vi "Display.vi"(8 "error in (no error)":errorcluster, 11 "DisplayTetrodes in":refnum<class "DisplayTetrodes.lvclass">) -> (0 "error out":errorcluster, 3 "DisplayTetrodes out":refnum<class "DisplayTetrodes.lvclass">)   [LabVIEW 2010, in "DisplayTetrodes.lvclass"]
uses:
  DisplayTetrodes.lvclass
  <vilib>/Analysis/3filter.llb/Filter Passband Type.ctl
  <vilib>/Analysis/2dsp.llb/Decimate (continuous, DBL).vi
  <vilib>/Analysis/3filter.llb/Butterworth Filter (DBL).vi
  Program Files/National Instruments/LabVIEW 2010/resource/objmgr/ni.dex.rc
  <vilib>/Analysis/NI_AALBase.lvlib
  <vilib>/Analysis/NI_AALPro.lvlib
panel:
  in  "Tab Control":enum32{"Connection", "Filter", "Display Params"}(tab)
  in  "Network Stream Writer IP":string(combo)
  out "Connected":bool
  out "Elems Left":i32(slide) scale=0.0..100.0
  in  "High Cutoff (Hz)":dbl=6000.0 format="%0.2f"
  in  "Low Cutoff (Hz)":dbl=600.0 format="%0.4f"
  in  "Filter Type":T1=enum."Bandpass"
  in  "FilterData":bool=TRUE
  in  "Decimation Factor":i32=4
  in  "Spacing":dbl=0.0001
  in  "Scale":dbl=1.0
  in  "DiodeScale":dbl=0.05
  out "Waveform Chart":waveform(dbl)[](graph)
  in  "STOP":bool
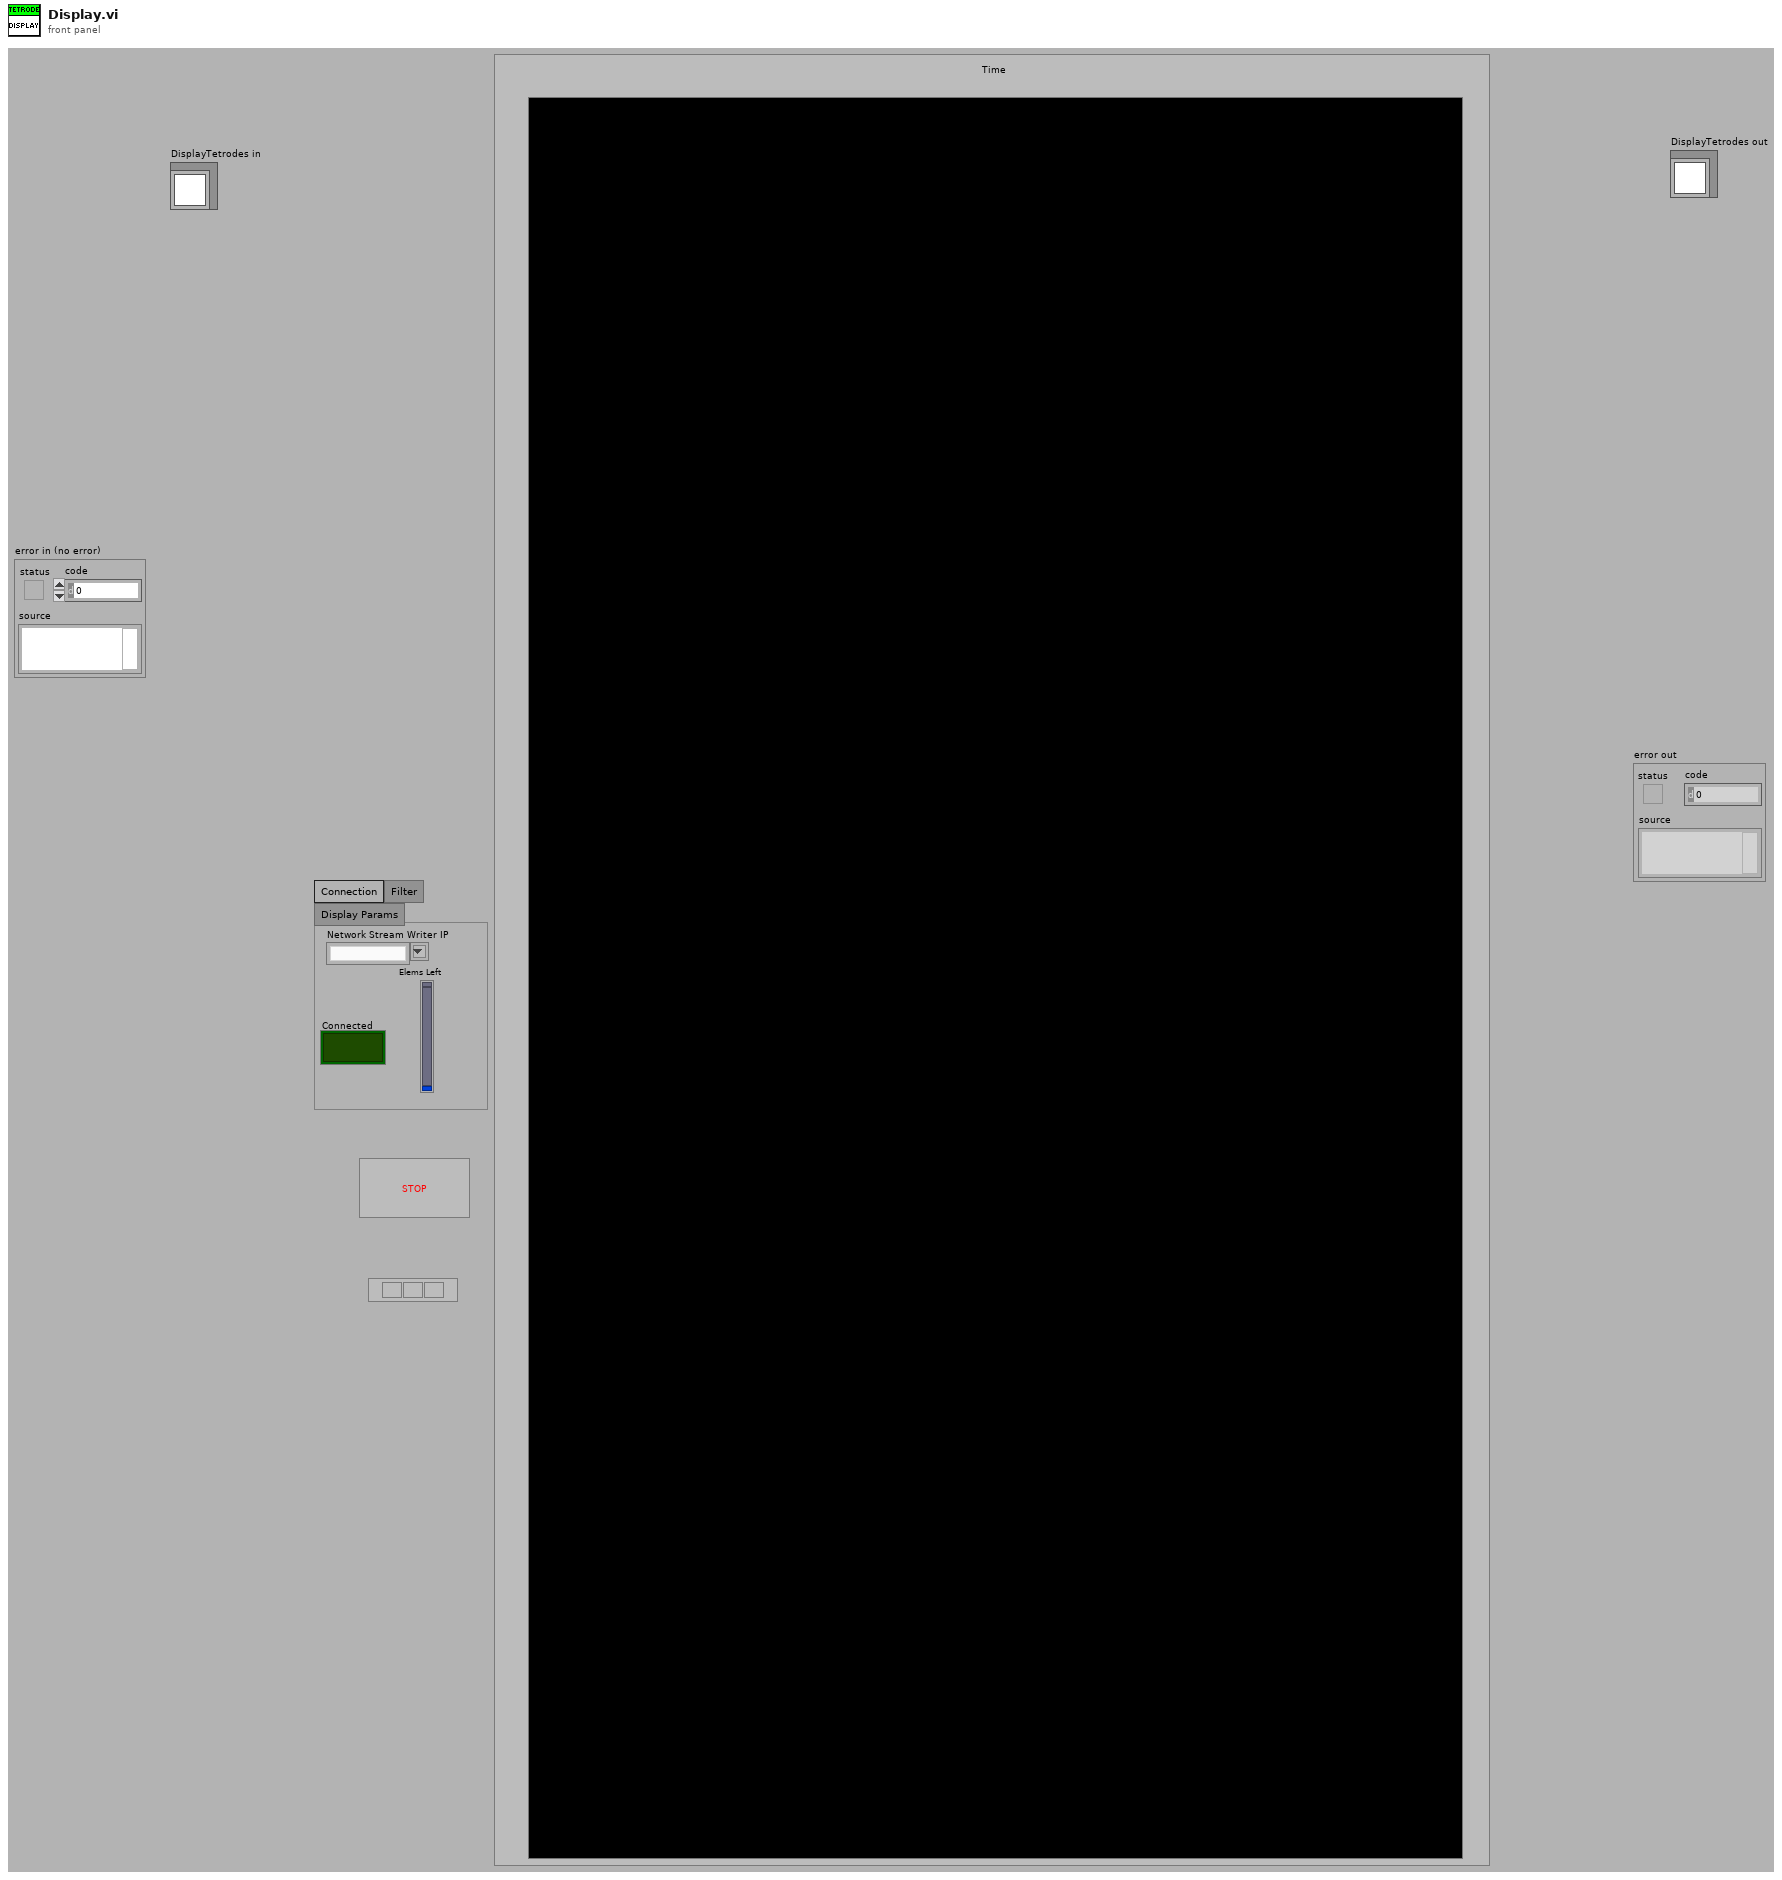
[diagram p1: front panel]
types:
  T1 = typedef "NI_AALBase.lvlib/Filter Passband Type.ctl" = enum32{"Lowpass", "Highpass", "Bandpass", "Bandstop"}
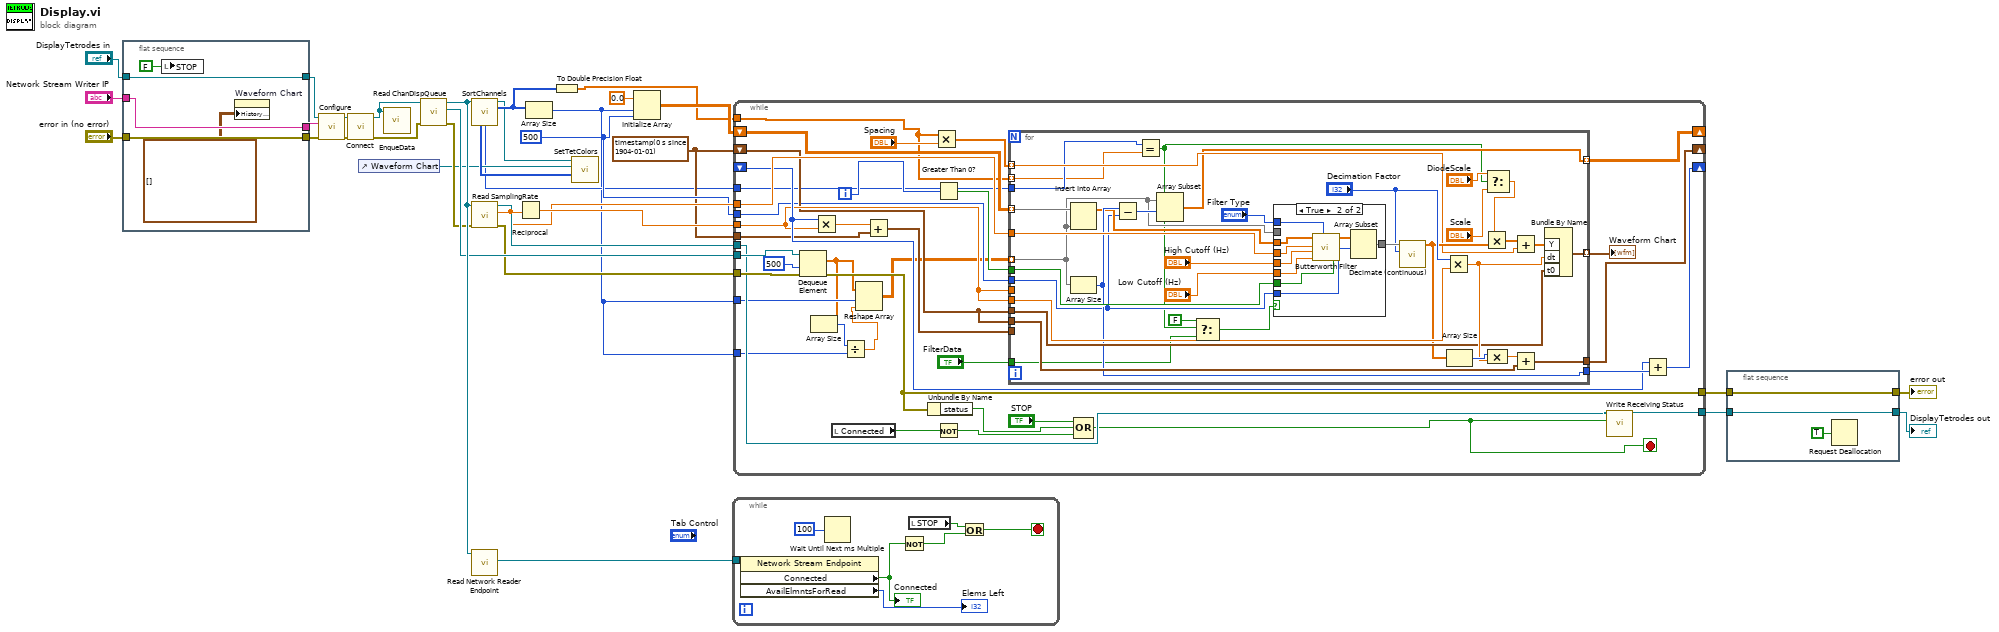
[diagram p0: block diagram]
diagram:
  w8 = timestamp(0 s since 1904-01-01)
  w9 = 500 ("y")
  n1 = flat-sequence {
    tunnel: "DisplayTetrodes in" -> [w37]
    tunnel: [w37] -> w17
    tunnel: "Network Stream Writer IP" -> [w36]
    tunnel: [w36] -> w15
    tunnel: "error in (no error)" -> [w35]
    tunnel: [w35] -> w13
    frame #0 {
      n2 = local write "STOP"(FALSE ("STOP")) -> ()
      n3 = property on="Waveform Chart" class="WFChart (strict)"("History Data"=waveform(dbl)[][] []) -> ()  [unwired: 2 in, 2 out]
    }
  }
  n4 = call-dynamic "Configure.vi"("error in (no error)"=w13, "Network Stream Writer IP"=w15, "DataReceiver in"=w17) -> ("error out"=w26:errorcluster, "DataReceiver out"=w28:refnum<class "DisplayTetrodes.lvclass">)  [unwired: 7 in]
  n5 = call-dynamic "Connect.vi"("error in (no error)"=w26, "DataReceiver in"=w28) -> ("error out"=w25:errorcluster, "DataReceiver out"=w27:refnum<class "DisplayTetrodes.lvclass">)  [unwired: 8 in]
  n6 = control-ref of="Waveform Chart"() -> (w3:refnum<vi>)
  n7 = call-dynamic "EnqueData.vi"("DataReceiver in"=w27) -> ()  [unwired: 9 in, 2 out]
  n8 = call-dynamic "Read ChanDispQueue.vi"("error in (no error)"=w25, "DataReceiver in"=w27) -> ("error out"=w30:errorcluster, "ChanDispQueue"=w31:refnum<queue>, "DataReceiver out"=w32:refnum<class "DisplayTetrodes.lvclass">)  [unwired: 7 in]
  n9 = call-dynamic "SortChannels.vi"("DisplayTetrodes in"=w32) -> ("DisplayTetrodes out"=w5:refnum<class "DisplayTetrodes.lvclass">, "reorderedChanNums"=w7:i32[], "unsortedTetNums"=w4:i32[], "reorderedDiodeChan"=w2:i32)  [unwired: 6 in, 5 out]
  n10 = call-dynamic "Read SamplingRate.vi"("error in (no error)"=w30, "DataReceiver in"=w32) -> ("error out"=w29:errorcluster, "SamplingRate"=w12:dbl, "DataReceiver out"=w24:refnum<class "DisplayTetrodes.lvclass">)  [unwired: 7 in]
  n11 = call-dynamic "Read Network Reader Endpoint.vi"("DataReceiver in"=w32) -> ("Network Stream Reader Endpoint"=w33:refnum<k21>)  [unwired: 8 in, 2 out]
  n12 = Reciprocal(x=w12) -> (1/x=w21:dbl)
  n13 = Array Size(array=w7) -> (size(s)=w1:i32)
  n14 = To Double Precision Float(number=w7) -> (double precision float=w6:dbl[])
  n15 = call-dynamic "SetTetColors.vi"("Unsorted Tet Nums"=w4, "WFChart Refnum"=w3, "DisplayTetrodes in"=w5) -> ()  [unwired: 7 in, 2 out]
  n16 = Initialize Array(0.0 ("element"), w1, w9) -> (w10:dbl[][])
  n17 = while {
    tunnel: w33 -> [w45]
    stop <- w44 stop-if-true
    n18 = property class="Network Stream Endpoint"(reference=w45) -> ("Connected"=w40:bool, "AvailElmntsForRead"=→"Elems Left":i32)  [unwired: 1 in, 2 out]
    "Connected" <- w40
    n19 = Wait Until Next ms Multiple(millisecond multiple=u32 100) -> ()  [unwired: 1 out]
    n20 = Not(x=w40) -> (.not. x?=w41:bool)
    n21 = local read "STOP"() -> (w42:bool)
    n22 = Or(x=w42, y=w41) -> (x .or. y?=w44:bool)
  }
  n23 = while {
    tunnel: w12 -> [w81]
    tunnel: [w73] -> w23
    tunnel: w31 -> [w78]
    tunnel: w29 -> [w77]
    tunnel: w24 -> [w71]
    tunnel: [w74] -> w20
    tunnel: w6 -> [w53]
    tunnel: w21 -> [w62]
    shift-right: [w67] -> _
    shift-left: _ -> [w66]
    tunnel: w8 -> [w64]
    shift-right: [w59] -> _
    shift-left: w8 -> [w60]
    shift-right: [w58] -> _
    shift-left: w10 -> [w57]
    tunnel: w9 -> [w56]
    tunnel: w2 -> [w54]
    tunnel: w1 -> [w51]
    tunnel: w1 -> [w49]
    i -> [w83]
    stop <- w52 stop-if-true
    n24 = Dequeue Element(queue=w78, timeout in ms (-1)=500, error in (no error)=w77) -> (element=w50:dbl[], error out=w73:errorcluster)  [unwired: 2 out]
    n25 = Array Size(array=w50) -> (size(s)=w48:i32)
    n26 = Multiply(x=w66, y=w62) -> (x*y=w65:dbl)
    n27 = local read "Connected"() -> (w70:bool)
    n28 = Divide(x=w48, y=w49) -> (x/y=w47:dbl)
    n29 = Reshape Array(w50, w51, w47) -> (w46:dbl[][])
    n30 = Add(x=w65, y=w64) -> (x+y=w63:timestamp)
    n31 = Unbundle By Name(w73) -> ("status"=w75:bool)
    n32 = Multiply(x=w53, y="Spacing") -> (x*y=w79:dbl[])
    n33 = Greater Than 0?(x=w83) -> (x > 0?=w82:bool)
    n34 = Not(x=w70) -> (.not. x?=w69:bool)
    n35 = for {
      tunnel: w46 -> [w95] mode=indexing
      tunnel: w82 -> [w116]
      tunnel: w81 -> [w117]
      tunnel: w79 -> [w102] mode=indexing
      tunnel: w62 -> [_]
      tunnel: [w100] -> w68
      tunnel: w63 -> [_]
      tunnel: w62 -> [w113]
      tunnel: w60 -> [w108]
      tunnel: [w107] -> w61 mode=indexing
      tunnel: w60 -> [w106]
      tunnel: [w105] -> w59
      tunnel: [w98] -> w58 mode=indexing
      tunnel: w57 -> [w97] mode=indexing
      tunnel: w56 -> [w94]
      tunnel: "FilterData" -> [w86]
      tunnel: w54 -> [w89]
      tunnel: w53 -> [w88] mode=indexing
      n36 = Insert Into Array(array=w97, new element=w95) -> (w96:dbl[])  [unwired: 1 in]
      n37 = Array Size(array=w95) -> (size(s)=w100:i32)
      n38 = Subtract(x=w100, y=w94) -> (x-y=w99:i32)
      n39 = Equal?(x=w89, y=w88) -> (x = y?=w87:bool)
      n40 = Array Subset(array=w95, index=w99) -> (w98:dbl[])  [unwired: 1 in]
      n41 = Select(t=FALSE, s=w87, f=w86) -> (s? t:f=w84:bool)
      n42 = case shown="True" w84 {
        tunnel: "High Cutoff (Hz)" -> [_ w128]
        tunnel: "Low Cutoff (Hz)" -> [_ w127]
        tunnel: w117 -> [_ w126]
        tunnel: w116 -> [_ w125]
        tunnel: "Filter Type" -> [_ w124]
        tunnel: [w119 w120] -> w114
        tunnel: w96 -> [_ w123]
        tunnel: w95 -> [w119 _]
        tunnel: w94 -> [_ w121]
        frame False {
        }
        frame True {
          n43 = call-poly <vilib>:"Butterworth Filter.vi"("init/cont (init:F)"=w125, "filter type"=w124, "low cutoff freq: fl"=w127, "high cutoff freq: fh"=w128, "sampling freq: fs"=w126, "X"=w123) -> ("Filtered X"=w122:dbl[])  [unwired: 2 in, 1 out]
          n44 = Array Subset(array=w122, index=w121) -> (w120:dbl[])  [unwired: 1 in]
        }
      }
      n45 = call-poly <vilib>:"Decimate (continuous).vi"("decimating factor"="Decimation Factor", "X"=w114) -> ("Decimated Array"=w103:dbl[])  [unwired: 8 in, 1 out]
      n46 = Multiply(x="Decimation Factor", y=w113) -> (x*y=w110:dbl)
      n47 = Array Size(array=w103) -> (size(s)=w112:i32)
      n48 = Select(t="DiodeScale", s=w87, f="Scale") -> (s? t:f=w90:dbl)
      n49 = Multiply(x=w90, y=w103) -> (x*y=w104:dbl[])
      n50 = Compound Arithmetic op=MULTIPLY(w112, w110) -> (w109:dbl)
      n51 = Add(x=w104, y=w102) -> (x+y=w101:dbl[])
      n52 = Add(x=w109, y=w108) -> (x+y=w105:timestamp)
      n53 = Bundle By Name("Y"=w101, "dt"=w110, "t0"=w106) -> (w107:waveform(dbl))  [unwired: 1 in]
    }
    "Waveform Chart" <- w61
    n54 = Compound Arithmetic op=OR("STOP", w75, w69) -> (w52:bool)
    n55 = call-dynamic "Write Receiving Status.vi"("Stop Reading"=w52, "DataReceiver in"=w71) -> ("DataReceiver out"=w74:refnum<class "DisplayTetrodes.lvclass">)  [unwired: 8 in, 1 out]
    n56 = Add(x=w66, y=w68) -> (x+y=w67:i32)
  }
  n57 = flat-sequence {
    tunnel: w23 -> [w131]
    tunnel: [w131] -> w22
    tunnel: w20 -> [w130]
    tunnel: [w130] -> w19
    frame #0 {
      n58 = Request Deallocation(TRUE ("flag")) -> ()
    }
  }
  "error out" <- w22
  "DisplayTetrodes out" <- w19
